vi "ReadTriggerScanNode.vi"(8 "Error In":errorcluster, 11 "Multiplexer Node In":refnum<k20>) -> (0 "Error Out":errorcluster, 2 "Trigger Scan Configuration":T1, 3 "Multiplexer Node Out":refnum<k20>)   [LabVIEW 2012]
uses:
  TriggerScanConfiguration.ctl
  driver/Public/Controls/ScanSource.ctl
  <vilib>/xml/NI_XML.lvlib
  driver/Keithley-7001.lvlib
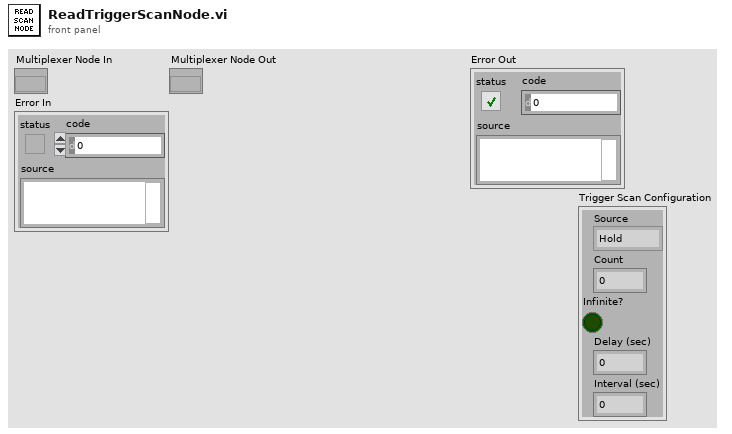
[diagram p1: front panel]
types:
  T1 = typedef "TriggerScanConfiguration.ctl" = cluster{"Source":T2, "Count":u32, "Infinite?":bool, "Delay (sec)":dbl, "Interval (sec)":dbl}
  T2 = typedef "Keithley-7001.lvlib/ScanSource.ctl" = enum16{"Hold", "Immediate", "Timer", "Manual", "Bus", "TLink", "External"}
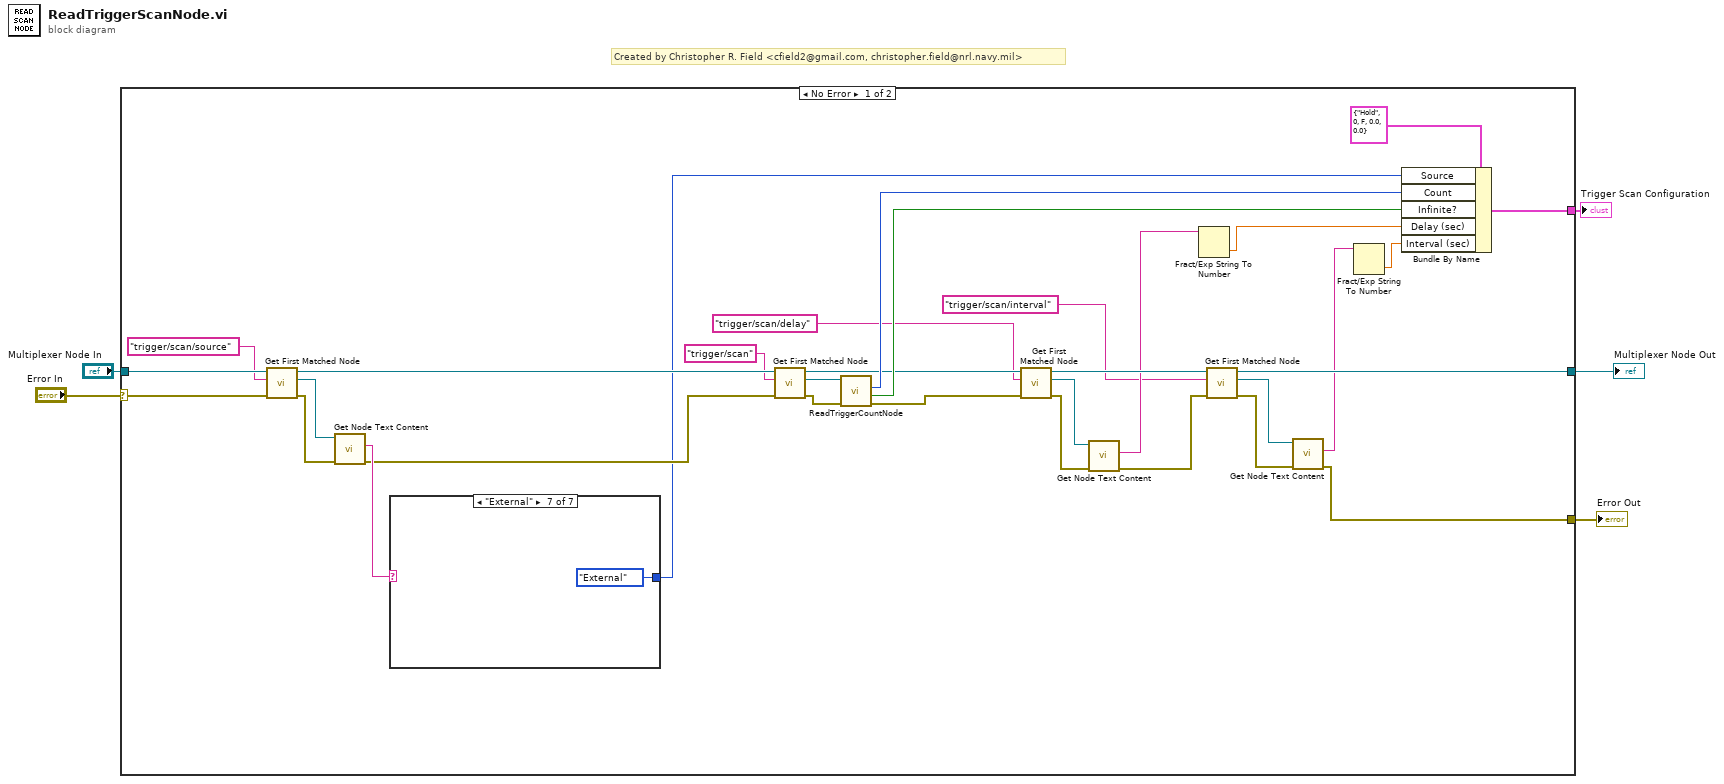
[diagram p0: block diagram]
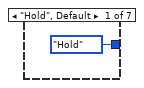
[diagram p2: hidden frame]
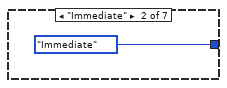
[diagram p3: hidden frame]
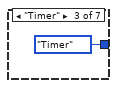
[diagram p4: hidden frame]
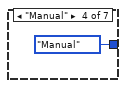
[diagram p5: hidden frame]
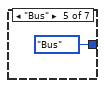
[diagram p6: hidden frame]
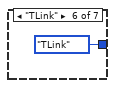
[diagram p7: hidden frame]
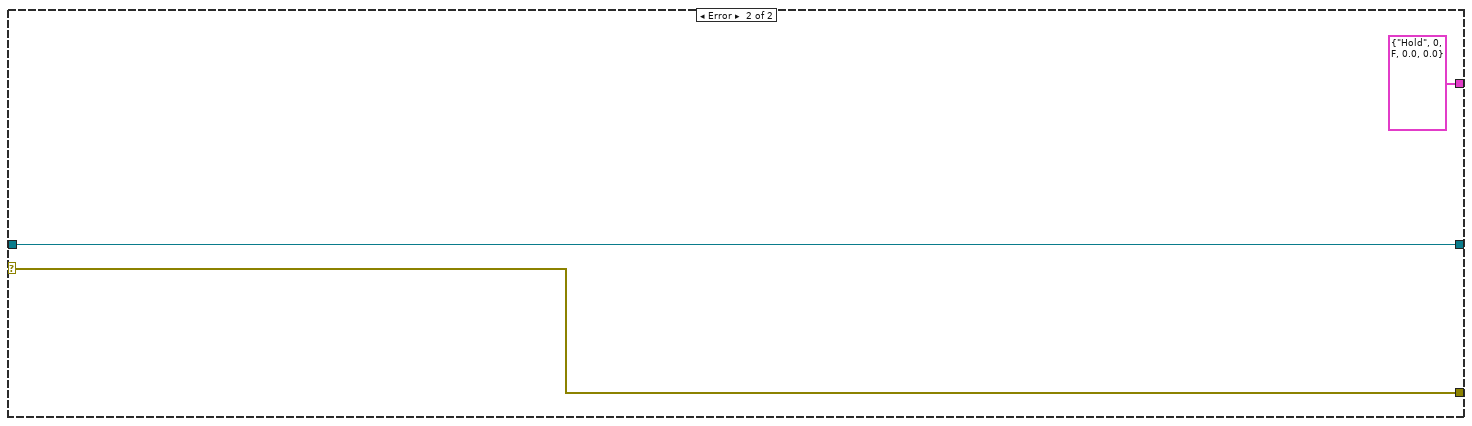
[diagram p8: hidden frame]
diagram:
  # "Created by Christopher R. Field <cfield2@gmail.com, christopher.field@nrl.navy.mil>"
  n1 = case shown="No Error" "Error In" {
    selector: "Error In" -> [w33 w46]
    tunnel: "Multiplexer Node In" -> [w37 w47]
    tunnel: [w12 w46] -> w3
    tunnel: [w16 w47] -> w2
    tunnel: [w7 T1 {"Source"=enum."Hold", "Count"=0, "Infinite?"=FALSE, "Delay (sec)"=0.0, "Interval (sec)"=0.0} ("Trigger Scan Configuration")] -> w1
    frame No Error {
      n2 = call <vilib>:"Get First Matched Node.vi"("error in (no error)"=w33, "XPath expression"="trigger/scan/source", "node in"=w37) -> ("error out"=w34:errorcluster, "node result"=w35:refnum<k20>, "node out"=w31:refnum<k20>)  [unwired: 6 in]
      n3 = call <vilib>:"Get Node Text Content.vi"("error in (no error)"=w34, "node in"=w35) -> ("error out"=w28:errorcluster, "node text"=w32:string)  [unwired: 7 in, 1 out]
      n4 = case shown="\"External\"" w32 {
        tunnel: [ScanSource."Hold" ("Source") ScanSource."Immediate" ("Source") ScanSource."Timer" ("Source") ScanSource."Manual" ("Source") ScanSource."Bus" ("Source") ScanSource."TLink" ("Source") ScanSource."External" ("Source")] -> w23
        frame "Hold", Default {
        }
        frame "Immediate" {
        }
        frame "Timer" {
        }
        frame "Manual" {
        }
        frame "Bus" {
        }
        frame "TLink" {
        }
        frame "External" {
        }
      }
      n5 = call <vilib>:"Get First Matched Node.vi"("error in (no error)"=w28, "XPath expression"="trigger/scan", "node in"=w31) -> ("error out"=w27:errorcluster, "node result"=w29:refnum<k20>, "node out"=w22:refnum<k20>)  [unwired: 6 in]
      n6 = call "ReadTriggerCountNode.vi"("Error In"=w27, "Trigger Node In"=w29) -> ("Error Out"=w21:errorcluster, "Infinite?"=w25:bool, "Count"=w26:u32)  [unwired: 6 in, 1 out]
      n7 = call <vilib>:"Get First Matched Node.vi"("error in (no error)"=w21, "XPath expression"="trigger/scan/delay", "node in"=w22) -> ("error out"=w18:errorcluster, "node result"=w19:refnum<k20>, "node out"=w17:refnum<k20>)  [unwired: 6 in]
      n8 = call <vilib>:"Get Node Text Content.vi"("error in (no error)"=w18, "node in"=w19) -> ("error out"=w15:errorcluster, "node text"=w11:string)  [unwired: 7 in, 1 out]
      n9 = Fract/Exp String To Number(string=w11) -> (number=w10:dbl)  [unwired: 3 in, 1 out]
      n10 = call <vilib>:"Get First Matched Node.vi"("error in (no error)"=w15, "XPath expression"="trigger/scan/interval", "node in"=w17) -> ("error out"=w13:errorcluster, "node result"=w14:refnum<k20>, "node out"=w16:refnum<k20>)  [unwired: 6 in]
      n11 = call <vilib>:"Get Node Text Content.vi"("error in (no error)"=w13, "node in"=w14) -> ("error out"=w12:errorcluster, "node text"=w9:string)  [unwired: 7 in, 1 out]
      n12 = Fract/Exp String To Number(string=w9) -> (number=w8:dbl)  [unwired: 3 in, 1 out]
      n13 = Bundle By Name(cluster=T1 {"Source"=enum."Hold", "Count"=0, "Infinite?"=FALSE, "Delay (sec)"=0.0, "Interval (sec)"=0.0} ("Trigger Scan Configuration"), "Source"=w23, "Count"=w26, "Infinite?"=w25, "Delay (sec)"=w10, "Interval (sec)"=w8) -> (w7:T1)
    }
    frame Error {
    }
  }
  "Error Out" <- w3
  "Multiplexer Node Out" <- w2
  "Trigger Scan Configuration" <- w1
